vi "_Split Calibration Table.vi"(0 "Calibration":dbl[][](array[numeric])) -> (1 "Mass":dbl[](array[numeric]), 2 "DAC":dbl[](array[numeric]))   [LabVIEW 2015]
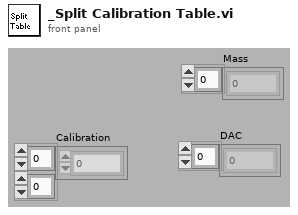
[diagram p1: front panel]
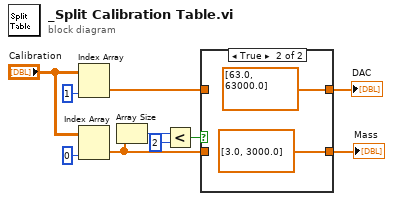
[diagram p0: block diagram]
diagram:
  n1 = Index Array(array="Calibration", index (col)=1 ("Index")) -> (element=w3:dbl[])  [unwired: 1 in]
  n2 = Index Array(array="Calibration", index (col)=0 ("Index")) -> (element=w4:dbl[])  [unwired: 1 in]
  n3 = Array Size(array=w4) -> (size(s)=w7:i32)
  n4 = Less?(x=w7, y=2) -> (x < y?=w5:bool)
  n5 = case shown="True" w5 {
    tunnel: w4 -> [w11 _]
    tunnel: w3 -> [w12 _]
    tunnel: [w11 dbl[] [3.0, 3000.0]] -> w2
    tunnel: [w12 dbl[] [63.0, 63000.0]] -> w1
    frame False {
    }
    frame True {
    }
  }
  "DAC" <- w1
  "Mass" <- w2
